vi "accum-array-size-resetable.vi"(6 "reset":bool, 11 "array":dbl[][](array[numeric])) -> (3 "accumulated-size":i32)   [LabVIEW 2017]
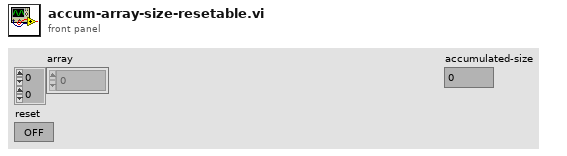
[diagram p1: front panel]
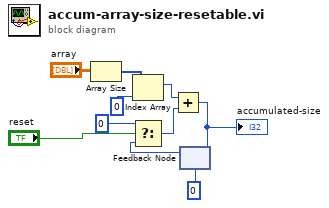
[diagram p0: block diagram]
diagram:
  n1 = Array Size(array="array") -> (size(s)=w8:i32[])
  n2 = Index Array(array=w8, index=0) -> (element=w7:i32)
  n3 = feedback #1(0) -> (w4:i32)
  n4 = Select(t=0, s="reset", f=w4) -> (s? t:f=w3:i32)
  n5 = Add(x=w7, y=w3) -> (x+y=w6:i32)
  "accumulated-size" <- w6
  n6 = feedback-in #1(w6) -> ()
